vi "Read Delta.vi"(8 "error in (no error)":errorcluster, 11 "Guidance in":refnum<class "Guidance.lvclass">) -> (0 "error out":errorcluster, 2 "Delta":T1, 3 "Guidance out":refnum<class "Guidance.lvclass">)   [LabVIEW 2014, in "Guidance Library.lvlib" / "Guidance.lvclass"]
uses:
  Guidance.lvclass
  <vilib>/Analysis/Matrix/Datatypes/RealMatrix.ctl
  Guidance.lvclass/Guidance.ctl
  <vilib>/Analysis/Matrix/NI_Matrix.lvlib
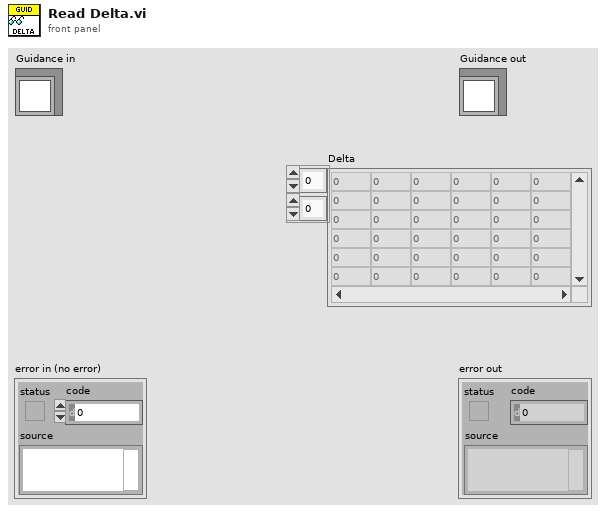
[diagram p1: front panel]
types:
  T1 = typedef "NI_Matrix.lvlib/RealMatrix.ctl" = dbl[][]
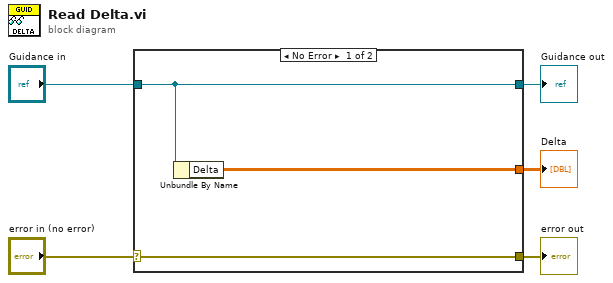
[diagram p0: block diagram]
diagram:
  n1 = case shown="No Error" "error in (no error)" {
    selector: "error in (no error)" -> [w8 w9]
    tunnel: [w8 w9] -> w4
    tunnel: [w7 w10] -> w2
    tunnel: "Guidance in" -> [w7 w10]
    tunnel: [w6 _] -> w1
    frame No Error {
      n2 = Unbundle By Name(w7) -> ("Delta"=w6:T1)
    }
    frame Error {
    }
  }
  "error out" <- w4
  "Guidance out" <- w2
  "Delta" <- w1
